vi "Material-Automation-LaunchAboutDialog.vi"(0 "Dialog Type":T1=enum."RequestStagingServer", 11 "error in":errorcluster) -> (15 "error out":errorcluster)   [LabVIEW 2013]
uses:
  Material-Automation-DialogType.ctl
panel:
  # "Inputs"
  # "Outputs"
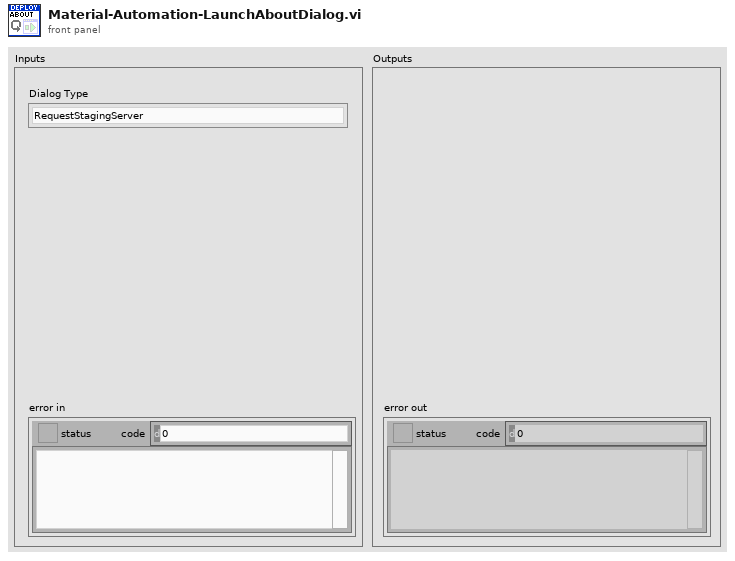
[diagram p1: front panel]
types:
  T1 = typedef "Material-Automation-DialogType.ctl" = enum16{"Registration", "Credits", "RequestStagingServer"}
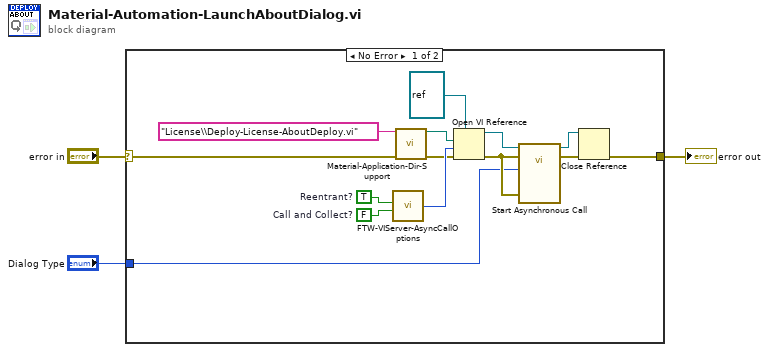
[diagram p0: block diagram]
diagram:
  n1 = case shown="No Error" "error in" {
    selector: "error in" -> [w13 w18]
    tunnel: [w17 w18] -> w3
    tunnel: "Dialog Type" -> [w4 _]
    frame No Error {
      w14 = FALSE  # Call and Collect?
      w15 = TRUE  # Reentrant?
      n2 = call "FTW-VIServer-AsyncCallOptions.vi"("Call and Collect?"=w14, "Reentrant?"=w15) -> ("Open VI Ref Options"=w16:i32)  [unwired: 4 in]
      n3 = call "Material-Application-Dir-Support.vi"("Support Resource Relative Filepath"="License\\Deploy-License-AboutDeploy.vi" ("Support VI Relative Filepath"), "error in"=w13) -> ("Support Filepath"=w11:path, "error out"=w12:errorcluster)  [unwired: 12 in]
      n4 = Open VI Reference(type specifier VI Refnum (for type only)=refnum<vi> refnum, vi path=w11, options=w16, error in (no error)=w12) -> (vi reference=w10:refnum<vi>, error out=w6:errorcluster)  [unwired: 2 in]
      n5 = call-by-ref "Start Asynchronous Call"(reference=w10, error in=w6, "Dialog Type"=w4, "error in"=w6) -> (reference out=w7:refnum<vi>, error out=w8:errorcluster)  [unwired: 13 in, 1 out]
      n6 = Close Reference(reference=w7, error in (no error)=w8) -> (error out=w17:errorcluster)
    }
    frame Error {
    }
  }
  "error out" <- w3
